vi "ACT_Loop.vi"() -> ()   [LabVIEW 2023, in "SwerveDrive_ACT_ts.lvlib"]
uses:
  SwerveDrive_ACT_ts.lvlib
  Cluster_CMD_ACT_Data.ctl
  Shared Code/TypeDefs/ENUM_CMD_Mode Select.ctl
  Shared Code/TypeDefs/Cluster_CMD_Direction Data.ctl
  Shared Code/TypeDefs/Cluster_Module Velocity-Direction-Rotations.ctl
  Shared Code/TypeDefs/Level_Velocity plus-minus 1.ctl
  Shared Code/TypeDefs/Dial_Compase heading unit circle CCW positive.ctl
  Shared Code/TypeDefs/Cluster_X-Y.ctl
  <vilib>/Rock Robotics/WPI/ThirdParty/REV Robotics/REVLib/Typedef/Spark MAX Control Type.ctl
  Type Defs/ENUM_Steer Mode Select.ctl
  Shared Code/TypeDefs/Cluster_Swerve 4 Steer and Velocity.ctl
  Shared Code/TypeDefs/Cluster_Swerve Actual Settings.ctl
  Shared Code/TypeDefs/Cluster_Module Actual Settings.ctl
  Shared Code/TypeDefs/Dial_Actual Direction.ctl
  ENUM_ACT_State.ctl
  <vilib>/Rock Robotics/WPI/MotorControl/WPI_MotorControlDeviceRef.ctl
  <vilib>/Rock Robotics/WPI/MotorControl/WPI_MotorControlType.ctl
  <vilib>/Rock Robotics/SystemInterfaces/DIO/FPGA_DIOPWMChannel.ctl
  <vilib>/Rock Robotics/WPI/PWM/WPI_PWMDeadband.ctl
  <vilib>/Rock Robotics/SystemInterfaces/DIO/FPGA_DIOChannel.ctl
  Shared Code/TypeDefs/ENUM_Module Position.ctl
  Type Defs/Cluster_Avoid Zone.ctl
  Shared Code/TypeDefs/Cluster_Config_Swerve Drive Parameters.ctl
  Type Defs/Cluster_Length and Width.ctl
  Shared Code/TypeDefs/Cluster_Config_Swerve_Steer Parm.ctl
  Shared Code/TypeDefs/Cluster_Config_Swerve_Drive Param.ctl
  <vilib>/Rock Robotics/WPI/ThirdParty/Phoenix-LabVIEW/CANCoder/Controls/CTRE_Phoenix_CANcoder_DeviceRef.ctl
  ENUM_ACT_Action.ctl
  RoboRIO Utilities/Global_STOP.vi
  Global_CMD_ACT_Data In.vi
  PigeonIMU/Global_SEN_Data Out.vi
  <vilib>/Rock Robotics/WPI/ThirdParty/Phoenix-LabVIEW/CANCoder/Get/CTRE_Phoenix_CANcoder_GetSensorData.vi
  Global_ACT_Data Out.vi
  PigeonIMU/PigeonIMU_SEN_ts.lvlib
panel:
  out "error out 2":errorcluster
  out "error out":errorcluster
  in  "OVERIDE Tab":enum32{"Teleop-Auto", "Move", "Stop"}(tab)
  in  "SEND CMD(Momentry)":bool
  in  "Rotation Reduction 1-0":dbl=0.5
  in  "Orientation Robot(t) Field(f)":bool=TRUE
  in  "Direction":T1 {"Rotate(Yaw) CCW 1 CW -1" scale=1.0..-1.0; "Traverse"."Angle" scale format="%.3f"; "Traverse"."Velocity" scale=-1.0..1.0 scale format="%.1f"}
  in  "Max Translation Speed (ft/sec)":dbl
  out "Cancoder Values":dbl[](array[numeric]) format="%#.6f"
  out "Steer values":dbl[](array[numeric]) format="%.6g"
  out "unit circ Steer values":dbl[](array[numeric]) format="%.6g"
  out "unit circ Cancoder values":dbl[](array[numeric]) format="%#.6f"
  out "Yaw":T4 scale format="%.3f"
  out "Swerve SET Actual":T5 {"Back Right"."Encoder" format="%.2f"; "Back Right"."Direction" scale format="%.3f"; "Back Right"."Velocity" format="%.2f"; "Back Left"."Encoder" format="%.2f"; "Back Left"."Direction" scale format="%.3f"; "Back Left"."Velocity" format="%.2f"; "Front Left"."Encoder" format="%.2f"; "Front Left"."Direction" scale format="%.3f"; "Front Left"."Velocity" format="%.2f"; "Front Right"."Encoder" format="%.2f"; "Front Right"."Direction" scale format="%.3f"; "Front Right"."Velocity" format="%.2f"}
  out "calc time":dbl
  out "Swerve Set":T8 {"Back Right"."Angle" scale format="%.3f"; "Back Right"."Velocity" scale=-1.0..1.0 scale format="%.1f"; "Back Left"."Angle" scale format="%.3f"; "Back Left"."Velocity" scale=-1.0..1.0 scale format="%.1f"; "Front Left"."Angle" scale format="%.3f"; "Front Left"."Velocity" scale=-1.0..1.0 scale format="%.1f"; "Front Right"."Angle" scale format="%.3f"; "Front Right"."Velocity" scale=-1.0..1.0 scale format="%.1f"}
  out "Max Velocity(RPM)":dbl=200.0
  out "Steer Mode":T9
  out "Max Velocity FPS":dbl=2.0
  out "Drive Control Mode":T10
  out "Input CMD":T11 {"Auto Angle" scale format="%.3f"; "Direction"."Rotate(Yaw) CCW 1 CW -1" scale=1.0..-1.0; "Direction"."Traverse"."Angle" scale format="%.3f"; "Direction"."Traverse"."Velocity" scale=-1.0..1.0 scale format="%.1f"}
  out "Cycle Time (S)":dbl format="%.3g"
  # "TeleOp or Auto Control"
  # "STOP"
  # "\"Front\" of Robot"
  # "X"
  # "+CCW"
  # "Y"
  # "(0,0)"
  # "\"Front\" of Robot"
  # "Index 1"
  # "Index 0"
  # "Index 3"
  # "Index 2"
  # "Right Hand Rule"
  # "X"
  # "+CCW"
  # "Y"
  # "(0,0)"
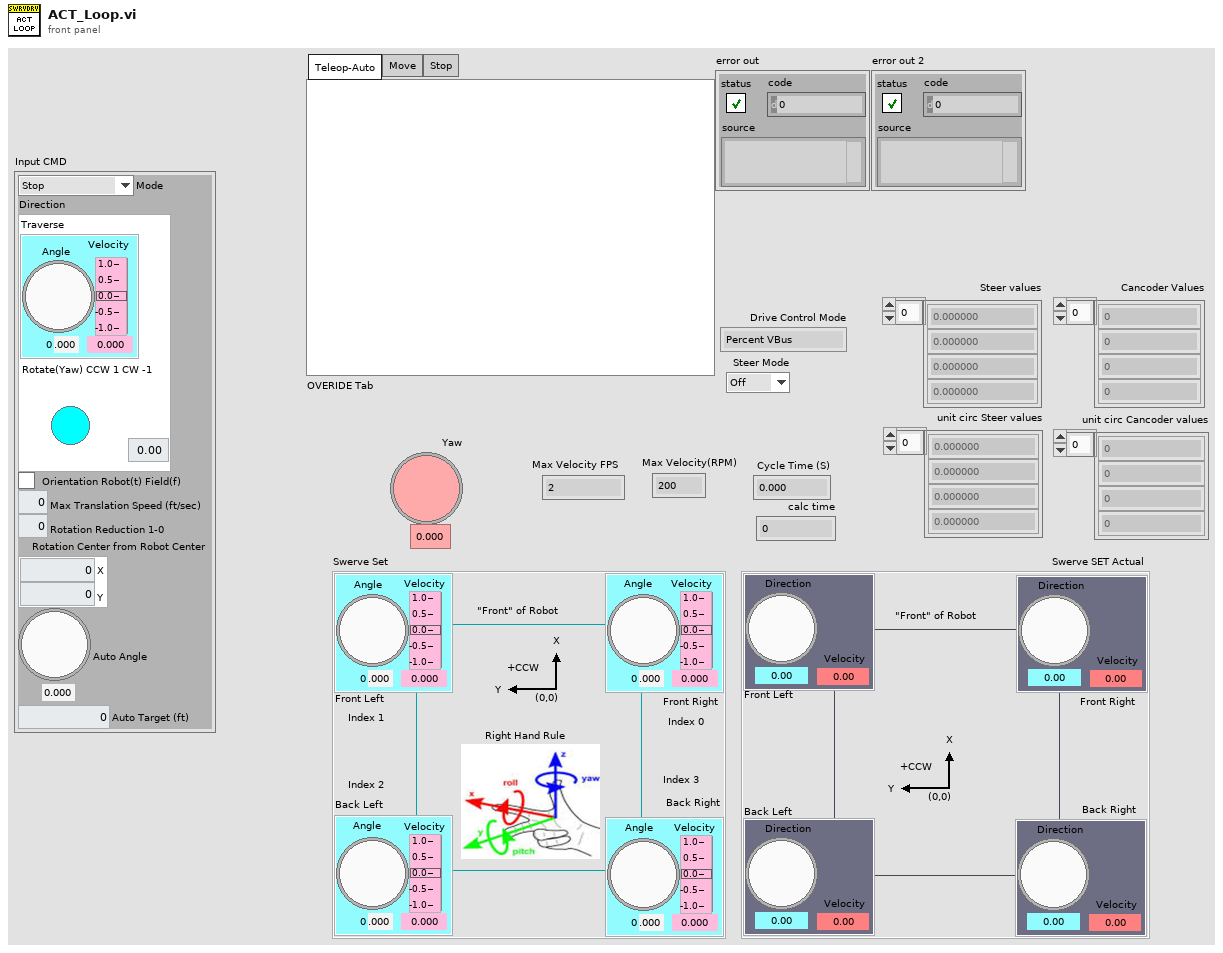
[diagram p1: front panel]
types:
  T1 = typedef "Cluster_CMD_Direction Data.ctl" = cluster{"Traverse":T2, "Rotate(Yaw) CCW 1 CW -1":dbl}
  T2 = typedef "Cluster_Module Velocity-Direction-Rotations.ctl" = cluster{"Velocity":T3, "Angle":T4, "Rotations Count":dbl}
  T3 = typedef "Level_Velocity plus-minus 1.ctl" = dbl
  T4 = typedef "Dial_Compase heading unit circle CCW positive.ctl" = dbl
  T5 = typedef "Cluster_Swerve Actual Settings.ctl" = cluster{"Front Right":T6, "Front Left":T6, "Back Left":T6, "Back Right":T6}
  T6 = typedef "Cluster_Module Actual Settings.ctl" = cluster{"Velocity":dbl, "Direction":T7, "Encoder":dbl}
  T7 = typedef "Dial_Actual Direction.ctl" = dbl
  T8 = typedef "Cluster_Swerve 4 Steer and Velocity.ctl" = cluster{"Front Right":T2, "Front Left":T2, "Back Left":T2, "Back Right":T2}
  T9 = typedef "ENUM_Steer Mode Select.ctl" = enum16{"Off", "Hold", "Steer"}
  T10 = typedef "Spark MAX Control Type.ctl" = enum16{"Percent VBus", "Voltage", "Velocity", "Position", "Smart Motion", "Current", "Smart Velocity"}
  T11 = typedef "SwerveDrive_ACT_ts.lvlib/Cluster_CMD_ACT_Data.ctl" = cluster{"Mode":T12, "Direction":T1, "Orientation Robot(t) Field(f)":bool, "Max Translation Speed (ft/sec)":dbl, "Rotation Reduction 1-0":dbl, "Rotation Center from Robot Center":T13, "Auto Angle":T4, "Auto Target (ft)":dbl}
  T12 = typedef "ENUM_CMD_Mode Select.ctl" = enum16{"Stop", "Move", "Turret Manual"}
  T13 = typedef "Cluster_X-Y.ctl" = cluster{"X":dbl, "Y":dbl}
  T14 = typedef "CTRE_Phoenix_CANcoder_DeviceRef.ctl" = cluster{"DeviceStatus":errorcluster, "Device Number":u8, "Handle":u64, "UsageFrame":u32, "Library Path":path}
  T15 = typedef "Cluster_Config_Swerve Drive Parameters.ctl" = cluster{"SwerveParam Ver":u64, "Frame":T16, "Steer":T17, "Drive":T18}
  T16 = typedef "Cluster_Length and Width.ctl" = cluster{"Length":dbl, "Width":dbl}
  T17 = typedef "Cluster_Config_Swerve_Steer Parm.ctl" = cluster{"CPR":dbl}
  T18 = typedef "Cluster_Config_Swerve_Drive Param.ctl" = cluster{"CPR":dbl, "RevMotor/Wheel":dbl, "Wheel Diameter (in)":dbl}
  T19 = typedef "Cluster_Avoid Zone.ctl" = cluster{"pos 1":dbl, "pos 2":dbl}
  T20 = typedef "ENUM_Module Position.ctl" = enum16{"Left-Front", "Right-Front", "Left-Back", "Right-Back"}
  T21 = typedef "WPI_MotorControlDeviceRef.ctl" = cluster{"DeviceStatus":errorcluster, "Type":T22, "PWM":cluster{"PWM Channel":T23, "DeadBand":T24}, "CAN":cluster{"Device Number":u8, "SetOutput VI Ref":variant, "GetOutput VI Ref":variant, "Enable VI Ref":variant, "Disable VI Ref":variant, "Data":variant}, "Invert":bool, "DIO PWM":cluster{"PWM \"Enable\" Channel":T23, "DIOChannel":T25, "PWM Rate":dbl}}
  T22 = typedef "WPI_MotorControlType.ctl" = enum16{"PWM", "CAN", "DIO PWM"}
  T23 = typedef "FPGA_DIOPWMChannel.ctl" = enum8{"PWM 0", "PWM 1", "PWM 2", "PWM 3", "PWM 4", "PWM 5", "PWM 6", "PWM 7", "PWM 8", "PWM 9", "PWM MXP 0", "PWM MXP 1", "PWM MXP 2", "PWM MXP 3", "PWM MXP 4", "PWM MXP 5", "PWM MXP 6", "PWM MXP 7", "PWM MXP 8", "PWM MXP 9", "Invalid"}
  T24 = typedef "WPI_PWMDeadband.ctl" = cluster{"Name":string, "maxPositivePwm":i32, "minPositivePwm":i32, "centerPwm":i32, "maxNegativePwm":i32, "minNegativePwm":i32, "angularRange":u16}
  T25 = typedef "FPGA_DIOChannel.ctl" = enum8{"DIO 0", "DIO 1", "DIO 2", "DIO 3", "DIO 4", "DIO 5", "DIO 6", "DIO 7", "DIO 8", "DIO 9", "DIO MXP 0", "DIO MXP 1", "DIO MXP 2", "DIO MXP 3", "DIO MXP 4", "DIO MXP 5", "DIO MXP 6", "DIO MXP 7", "DIO MXP 8", "DIO MXP 9", "DIO MXP 10", "DIO MXP 11", "DIO MXP 12", "DIO MXP 13", "DIO MXP 14", "DIO MXP 15", "SPI Port CS1", "SPI Port CS2", "SPI Port CS3", "SPI Port MISO", "SPI Port MOSI", "Invalid"}
  T26 = typedef "SwerveDrive_ACT_ts.lvlib/ENUM_ACT_State.ctl" = enum16{"Startup", "Stopping", "Moving", "Shutdown"}
  T27 = typedef "SwerveDrive_ACT_ts.lvlib/ENUM_ACT_Action.ctl" = enum16{"No Action", "Reset Time", "Reset All", "2 Pos Set Direction", "2 Pos Set Speed", "Record Data", "Set Move from Values", "Reset Steer to Absolute"}
  T28 = cluster{"Motor List":T20[], "Drive Refs":T21[], "Steer Refs":T21[], "State":T26, "Previous State":T26, "Current Time":timestamp, "Previous Time":timestamp, "Start Time":timestamp, "Target Time (ms)":u32, "Cycle Time(S)":dbl, "ACT Input":T11, "Drive Control Mode":T10, "Drive PID Slot":i32, "Steer Position Values":dbl[], "Drive Velocity Values":dbl[], "Steer Position Times":dbl[], "Drive Velocity Times":dbl[], "Stream":bool, "Drive Output Times":dbl[], "Drive Output Values":dbl[], "Zero Start Steer Positions":dbl[], "Steer Mode":T9, "Max Velocity RPM":dbl, "Avoid Zone":T19, "Swerve Set":T8, "calc Start Time":dbl, "Compass Heading":T4, "Swerve Config ":T15, "Team Folder":path, "Steer Output Times":dbl[], "Can Coder Refs":T14[], "Can Coder Output postions":dbl[]}
  T29 = typedef "Cluster_Unity Yaw-Pitch-Roll.ctl" = cluster{"Yaw":T4, "Pitch":T4, "Roll":T4}
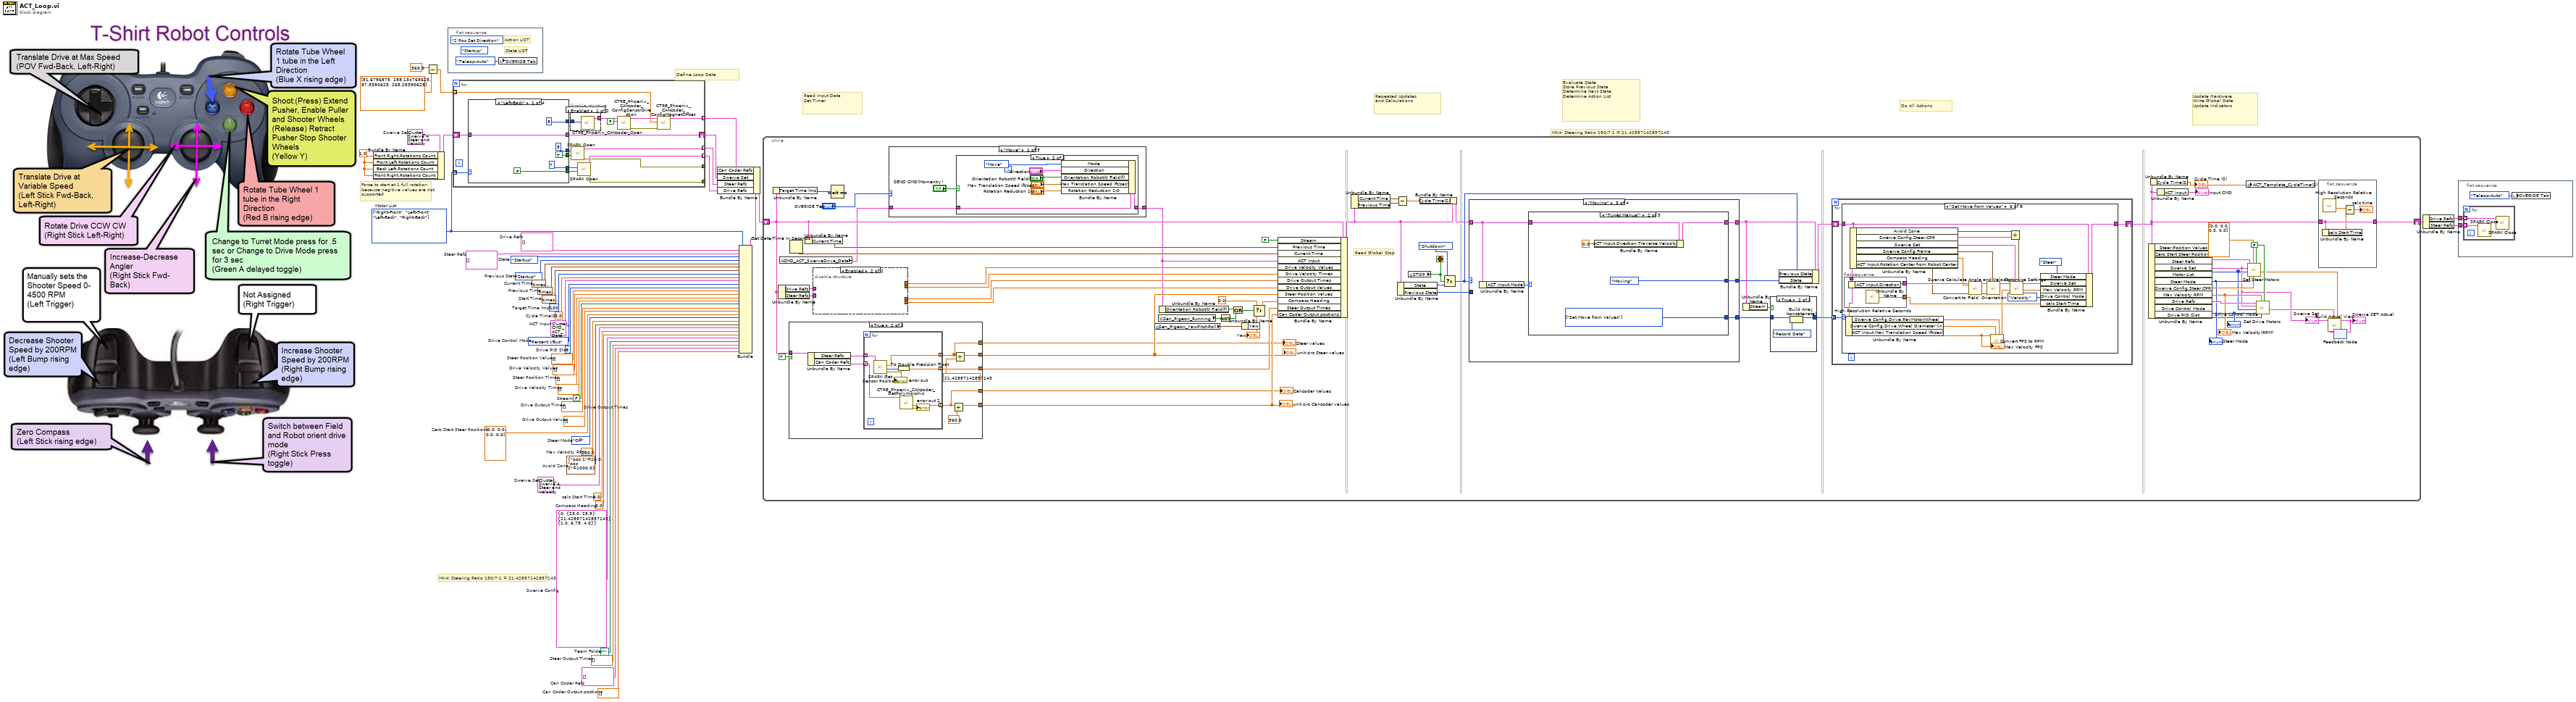
[diagram p0: block diagram]
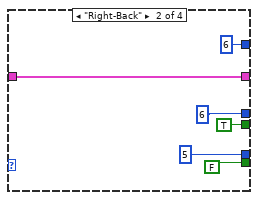
[diagram p3: hidden frame]
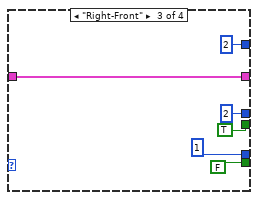
[diagram p4: hidden frame]
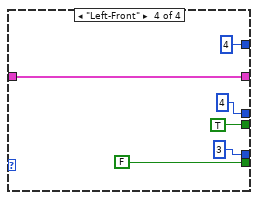
[diagram p5: hidden frame]
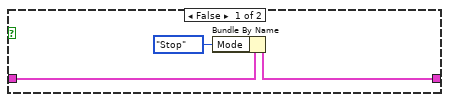
[diagram p6: hidden frame]
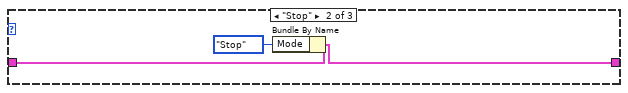
[diagram p7: hidden frame]
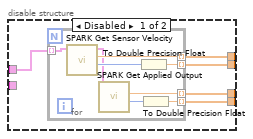
[diagram p9: hidden frame]
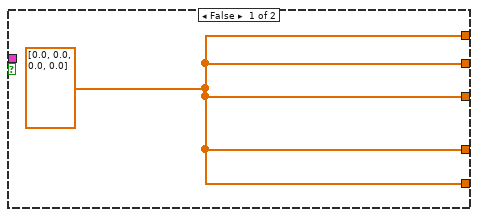
[diagram p10: hidden frame]
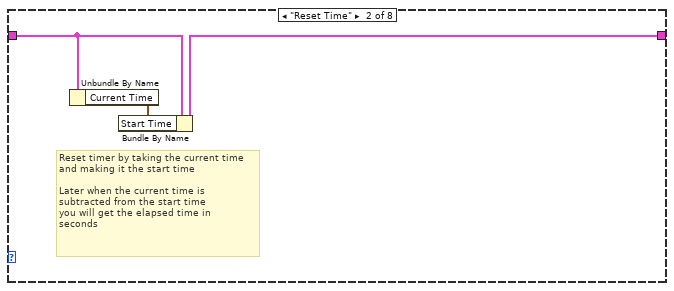
[diagram p13: hidden frame]
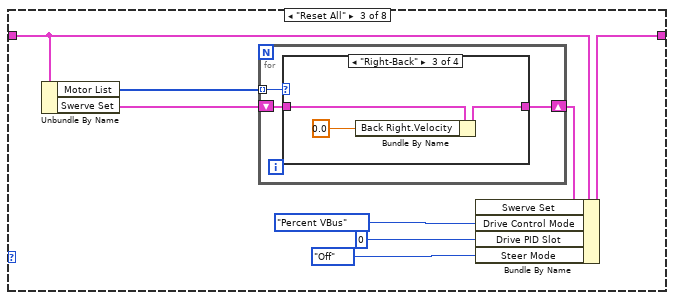
[diagram p14: hidden frame]
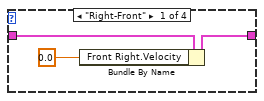
[diagram p15: hidden frame]
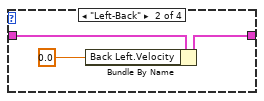
[diagram p16: hidden frame]
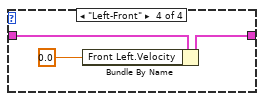
[diagram p17: hidden frame]
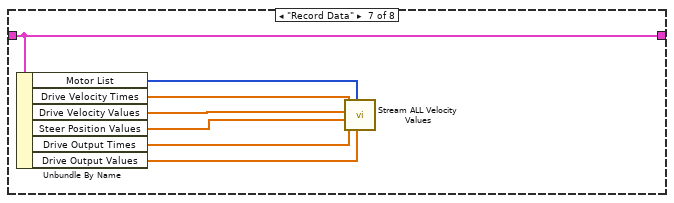
[diagram p20: hidden frame]
diagram:
  w4 = 1.0
  w8 = dbl[] []  # Can Coder Output postions
  w10 = T14[] []  # Can Coder Refs
  w11 = dbl[] []  # Steer Output Times
  (unwired) dbl[] []  # Drive Output Times
  w12 = path ""  # Team Folder
  w13 = T15 {"SwerveParam Ver"=0, "Frame"={"Length"=23.0, "Width"=25.5}, "Steer"={"CPR"=21.42857142857143}, "Drive"={"CPR"=1.0, "RevMotor/Wheel"=6.75, "Wheel Diameter (in)"=4.0}}  # Swerve Config
  w14 = T4 0.0  # Compass Heading
  w15 = 0.0  # calc Start Time
  w6 = T8 {"Front Right"={"Velocity"=0.0, "Angle"=0.0, "Rotations Count"=0.0}, "Front Left"={"Velocity"=0.0, "Angle"=0.0, "Rotations Count"=0.0}, "Back Left"={"Velocity"=0.0, "Angle"=0.0, "Rotations Count"=0.0}, "Back Right"={"Velocity"=0.0, "Angle"=0.0, "Rotations Count"=0.0}}  # Swerve Set
  w17 = T8 {"Front Right"={"Velocity"=0.0, "Angle"=0.0, "Rotations Count"=0.0}, "Front Left"={"Velocity"=0.0, "Angle"=0.0, "Rotations Count"=0.0}, "Back Left"={"Velocity"=0.0, "Angle"=0.0, "Rotations Count"=0.0}, "Back Right"={"Velocity"=0.0, "Angle"=0.0, "Rotations Count"=0.0}}  # Swerve Set
  w18 = T19 {"pos 1"=20.0, "pos 2"=1000.0}  # Avoid Zone
  w19 = T20[] [enum."Right-Front", enum."Left-Front", enum."Left-Back", enum."Right-Back"] items=["Left-Front", "Right-Front", "Left-Back", "Right-Back"]  # Motor List
  w20 = 200.0  # Max Velocity RPM
  w21 = ENUM_Steer_Mode_Select."Off"  # Steer Mode
  w22 = dbl[] [0.0, 0.0, 0.0, 0.0]  # Zero Start Steer Positions
  w23 = dbl[] []  # Drive Output Values
  w24 = dbl[] []  # Drive Output Times
  w25 = FALSE  # Stream
  w26 = dbl[] []  # Drive Velocity Times
  w27 = dbl[] []  # Steer Position Times
  w28 = dbl[] []  # Drive Velocity Values
  w29 = dbl[] []  # Steer Position Values
  w32 = 0  # Drive PID Slot
  w33 = Spark_MAX_Control_Type."Percent VBus"  # Drive Control Mode
  w37 = T21[] []  # Drive Refs
  w38 = T21[] []  # Steer Refs
  w40 = 0.0  # Cycle Time(S)
  w41 = ENUM_ACT_State."Startup"  # Previous State
  w42 = timestamp(0 s since 1904-01-01)  # Previous Time
  w43 = u32 100  # Target Time (ms)
  w44 = T11 {"Mode"=enum."Stop", "Direction"={"Traverse"={"Velocity"=0.0, "Angle"=0.0, "Rotations Count"=0.0}, "Rotate(Yaw) CCW 1 CW -1"=0.0}, "Orientation Robot(t) Field(f)"=FALSE, "Max Translation Speed (ft/sec)"=0.0, "Rotation Reduction 1-0"=0.0, "Rotation Center from Robot Center"={"X"=0.0, "Y"=0.0}, "Auto Angle"=0.0, "Auto Target (ft)"=0.0}  # ACT Input
  w45 = timestamp(0 s since 1904-01-01)  # Start Time
  w46 = timestamp(0 s since 1904-01-01)  # Current Time
  w47 = ENUM_ACT_State."Startup"  # State
  # "Force to start at 1 full rotation\nbecause negitive values are not\nsupported"
  # "MK4i Steering Ratio 150/7:1 = 21.42857142857143"
  # "MK4i Steering Ratio 150/7:1 = 21.42857142857143"
  # "Define Loop Data"
  # "Repeated Updates\nand Calculations"
  # "Read Input Data\nSet Timer"
  # "Evaluate State\nStore Previous State\nDetermine Next State\nDetermine Action List"
  # "Do All Actions"
  # "Update Hardware\nWrite Global Data\nUpdate Indicators"
  n1 = Bundle By Name(cluster=w6, "Front Right.Rotations Count"=w4, "Front Left.Rotations Count"=w4, "Back Left.Rotations Count"=w4, "Front Right.Rotations Count"=w4) -> (w5:T8)
  n2 = Subtract(x=360.0, y=dbl[] [51.6796875, 258.134765625, 87.5390625, 265.25390625] ("Cancoder Values")) -> (x-y=w1:dbl[])
  n3 = flat-sequence {
    frame #0 {
      (unwired) ENUM_ACT_State."Startup" ("State")
      (unwired) ENUM_ACT_Action."2 Pos Set Direction" ("Action")
      # "State LIST"
      # "Action LIST"
      n4 = local write "OVERIDE Tab"(enum32{"Teleop-Auto", "Move", "Stop"}."Teleop-Auto" ("OVERIDE Tab")) -> ()
    }
  }
  n5 = for {
    tunnel: w19 -> [w66] mode=indexing
    tunnel: [w60] -> w7 mode=indexing
    tunnel: [w63] -> w34 mode=indexing
    shift-right: [w64] -> w16
    shift-left: w5 -> [w65]
    tunnel: [w62] -> _
    tunnel: [w51] -> w9 mode=indexing
    tunnel: [w55] -> _
    tunnel: w1 -> [w49] mode=indexing
    n6 = case shown="\"Left-Back\"" w66 {
      tunnel: [FALSE ("Invert") FALSE ("Invert") FALSE ("Invert") FALSE ("Invert")] -> w61
      tunnel: [u8 7 ("unsigned 8bit integer") u8 5 ("unsigned 8bit integer") u8 1 ("unsigned 8bit integer") u8 3 ("unsigned 8bit integer")] -> w59
      tunnel: w65 -> [w69 w75 w81 w87]
      tunnel: [w69 w75 w81 w87] -> w64
      tunnel: [u8 8 ("Device Number") u8 6 ("Device Number") u8 2 ("Device Number") u8 4 ("Device Number")] -> w58
      tunnel: [TRUE ("Invert") TRUE ("Invert") TRUE ("Invert") TRUE ("Invert")] -> w57
      tunnel: [u8 8 ("Device Number") u8 6 ("Device Number") u8 2 ("Device Number") u8 4 ("Device Number")] -> w56
      frame "Left-Back" {
      }
      frame "Right-Back" {
      }
      frame "Right-Front" {
      }
      frame "Left-Front" {
      }
    }
    n7 = disable-structure shown="Enabled" {
      disable-tunnel: [w68 _] -> w54
      disable-tunnel: w56 -> [w67 _]
      frame Enabled {
        n8 = call <vilib>:"CTRE_Phoenix_CANcoder_Open.vi"("Device Number"=w67) -> ("CTRE_CANcoder_DeviceRef"=w68:T14)  [unwired: 9 in, 1 out]
      }
      frame Disabled {
      }
    }
    n9 = call <vilib>:"SPARK Open.vi"("Invert"=w57, "Device Number"=w58) -> ("error out"=w55:errorcluster, "MotorControlDeviceRef"=w60:T21)  [unwired: 8 in]
    n10 = call <vilib>:"SPARK Open.vi"("Invert"=w61, "Device Number"=w59) -> ("error out"=w62:errorcluster, "MotorControlDeviceRef"=w63:T21)  [unwired: 8 in]
    n11 = call <vilib>:"CTRE_Phoenix_CANcoder_ConfigSensorDirection.vi"("Sensor Direction"=FALSE, "CTRE_CANcoder_DeviceRef"=w54) -> ("error out"=w50:errorcluster, "CTRE_CANcoder_DeviceRef"=w52:T14)  [unwired: 8 in]
    n12 = call <vilib>:"CTRE_Phoenix_CANcoder_ConfigMagnetOffset.vi"("error in"=w50, "Magnet Offset (Degrees)"=w49, "CTRE_CANcoder_DeviceRef"=w52) -> ("CTRE_CANcoder_DeviceRef"=w51:T14)  [unwired: 7 in, 1 out]
  }
  n13 = Bundle("Motor List"=w19, "Drive Refs"=w37, "Steer Refs"=w38, "State"=w47, "Previous State"=w41, "Current Time"=w46, "Previous Time"=w42, "Start Time"=w45, "Target Time (ms)"=w43, "Cycle Time(S)"=w40, "ACT Input"=w44, "Drive Control Mode"=w33, "Drive PID Slot"=w32, "Steer Position Values"=w29, "Drive Velocity Values"=w28, "Steer Position Times"=w27, "Drive Velocity Times"=w26, "Stream"=w25, "Drive Output Times"=w24, "Drive Output Values"=w23, "Zero Start Steer Positions"=w22, "Steer Mode"=w21, "Max Velocity RPM"=w20, "Avoid Zone"=w18, "Swerve Set"=w17, "calc Start Time"=w15, "Compass Heading"=w14, "Swerve Config"=w13, "Team Folder"=w12, "Steer Output Times"=w11, "Can Coder Refs"=w10, "Can Coder Output postions"=w8) -> (w36:T28)  [unwired: 1 in]
  n14 = Bundle By Name(cluster=w36, "Can Coder Refs"=w9, "Swerve Set"=w16, "Steer Refs"=w7, "Drive Refs"=w34) -> (w35:T28)
  n15 = while {
    shift-right: [w100] -> w39
    shift-left: w35 -> [w127]
    stop <- w152 stop-if-true
    w116 = FALSE
    # "Read Global Stop"
    n16 = Unbundle By Name(w127) -> ("Target Time (ms)"=w149:u32)
    n17 = Unbundle By Name(w127) -> ("Drive Refs"=w126:T21[], "Steer Refs"=w99:T21[])
    n18 = global read "Global_CMD_ACT_Data In.vi" "CMD_ACT_SwerveDrive_Data"() -> (w96:T11)
    n19 = case shown="True" TRUE {
      tunnel: [w190 w194] -> w102
      tunnel: w127 -> [_ w200]
      tunnel: [w190 w195] -> w101
      tunnel: [w190 w197] -> w103
      tunnel: [w190 w192] -> w98
      tunnel: [w190 w191] -> w97
      frame False {
        w190 = dbl[] [0.0, 0.0, 0.0, 0.0]
      }
      frame True {
        n20 = Unbundle By Name(w200) -> ("Steer Refs"=w198:T21[], "Can Coder Refs"=w199:T14[])
        n21 = for {
          tunnel: [w204] -> w192 mode=indexing
          tunnel: [w207] -> w195 mode=indexing
          tunnel: w199 -> [w203] mode=indexing
          tunnel: [w206] -> w191 mode=indexing
          tunnel: w198 -> [w205] mode=indexing
          n22 = call <vilib>:"SPARK Get Sensor Position.vi"("MotorControlDevRef in"=w205) -> ("error out"=→"error out":errorcluster, "Timestamp"=w208:u32, "Sensor Position"=w204:dbl)  [unwired: 7 in, 1 out]
          n23 = To Double Precision Float(number=w208) -> (double precision float=w207:dbl)
          n24 = call-poly <vilib>:"CTRE_Phoenix_CANcoder_GetPolymorphic.vi"("CTRE_CANcoder_DeviceRef"=w203) -> ("Absolute Position"=w206:dbl, "error out"=→"error out 2":errorcluster)  [unwired: 10 in, 3 out]
        }
        n25 = Divide(x=w191, y=360.0 ("Absolute Position")) -> (x/y=w197:dbl[])
        n26 = Divide(x=w192, y=21.42857142857143 ("Absolute Position")) -> (x/y=w194:dbl[])
      }
    }
    "unit circ Cancoder values" <- w103
    "unit circ Steer values" <- w102
    "Steer values" <- w98
    "Cancoder Values" <- w97
    n27 = Get Date/Time In Seconds() -> (seconds since 1Jan1904=w155:timestamp)
    n28 = Unbundle By Name(w127) -> ("Current Time"=w148:timestamp)
    n29 = disable-structure shown="Enabled" {
      disable-tunnel: [w177 _] -> w136
      disable-tunnel: [w176 _] -> w135
      disable-tunnel: [w175 _] -> w133
      disable-tunnel: [w174 _] -> w132
      disable-tunnel: w126 -> [w173 _]
      disable-tunnel: w99 -> [_ _]
      frame Disabled {
        n30 = for {
          tunnel: w173 -> [w183] mode=indexing
          tunnel: [w182] -> w177 mode=indexing
          tunnel: [w185] -> w176 mode=indexing
          tunnel: [w179] -> w175 mode=indexing
          tunnel: [w184] -> w174 mode=indexing
          n31 = call <vilib>:"SPARK Get Sensor Velocity.vi"("MotorControlDevRef in"=w183) -> ("Timestamp"=w181:u32, "Sensor Velocity"=w182:dbl, "MotorControlDevRef out"=w180:T21)  [unwired: 7 in, 1 out]
          n32 = call <vilib>:"SPARK Get Applied Output.vi"("MotorControlDevRef in"=w180) -> ("Timestamp"=w178:u32, "Applied Output"=w179:dbl)  [unwired: 7 in, 2 out]
          n33 = To Double Precision Float(number=w181) -> (double precision float=w185:dbl)
          n34 = To Double Precision Float(number=w178) -> (double precision float=w184:dbl)
        }
      }
      frame Enabled {
      }
    }
    n35 = Wait (ms)(milliseconds to wait=w149) -> ()  [unwired: 1 out]
    n36 = case shown="\"Move\"" "OVERIDE Tab" {
      tunnel: w96 -> [w157 w171 w172]
      tunnel: [w156 w170 w172] -> w95
      frame "Move" {
        n37 = case shown="True" "SEND CMD(Momentry)" {
          tunnel: w157 -> [w161 w168]
          tunnel: [w160 w167] -> w156
          frame False {
            n38 = Bundle By Name(cluster=w161, "Mode"=ENUM_CMD_Mode_Select."Stop") -> (w160:T11)
          }
          frame True {
            n39 = Bundle By Name(cluster=w168, "Mode"=ENUM_CMD_Mode_Select."Move", "Direction"="Direction", "Orientation Robot(t) Field(f)"="Orientation Robot(t) Field(f)", "Max Translation Speed (ft/sec)"="Max Translation Speed (ft/sec)", "Rotation Reduction 1-0"="Rotation Reduction 1-0") -> (w167:T11)
          }
        }
      }
      frame "Stop" {
        n40 = Bundle By Name(cluster=w171, "Mode"=ENUM_CMD_Mode_Select."Stop") -> (w170:T11)
      }
      frame "Teleop-Auto" {
      }
    }
    n41 = global read "Global_SEN_Data Out.vi" "Sen_Pigeon_YawPitchRoll"() -> (w110:T29)
    n42 = global read "Global_SEN_Data Out.vi" "Sen_Pigeon_Running"() -> (w106:bool)
    n43 = Unbundle By Name(w95) -> ("Orientation Robot(t) Field(f)"=w112:bool)
    n44 = Not(x=w106) -> (.not. x?=w105:bool)
    n45 = Or(x=w112, y=w105) -> (x .or. y?=w107:bool)
    n46 = Unbundle By Name(w110) -> ("Yaw"=w109:T4)
    "Yaw" <- w109
    n47 = Select(t=T4 0.0, s=w107, f=w109) -> (s? t:f=w111:T4)
    n48 = Bundle By Name(cluster=w127, "Stream"=FALSE, "Previous Time"=w148, "Current Time"=w155, "ACT Input"=w95, "Drive Velocity Values"=w136, "Drive Velocity Times"=w135, "Drive Output Times"=w133, "Drive Output Values"=w132, "Steer Position Values"=w102, "Compass Heading"=w111, "Steer Output Times"=w101, "Can Coder Output postions"=w103) -> (w143:T28)
    n49 = Unbundle By Name(w143) -> ("Current Time"=w144:timestamp, "Previous Time"=w145:timestamp)
    n50 = Subtract(x=w144, y=w145) -> (x-y=w141:dbl)
    n51 = Unbundle By Name(w143) -> ("State"=w150:T26, "Previous State"=w147:T26)
    n52 = global read "Global_STOP.vi" "STOP"() -> (w152:bool)
    n53 = Bundle By Name(cluster=w143, "Cycle Time(S)"=w141) -> (w142:T28)
    n54 = Select(t=ENUM_ACT_State."Shutdown" ("State"), s=w152, f=w150) -> (s? t:f=w146:T26)
    n55 = case shown="\"Moving\"" w146 {
      tunnel: w142 -> [w288 w295 w307 w323]
      tunnel: [w290 w296 w308 w323] -> w131
      tunnel: [ENUM_ACT_State."Moving" ("State") w297 w309 ENUM_ACT_State."Shutdown" ("State")] -> w153
      tunnel: [w292 w293 w305 w321] -> w129
      tunnel: w147 -> [_ _ _ _]
      frame "Startup" {
        w292 = T27[] [enum."Reset Steer to Absolute", enum."Reset Time", enum."Reset All", enum."Reset Steer to Absolute"] items=["No Action", "Reset Time", "Reset All", "2 Pos Set Direction", "2 Pos Set Speed", "Record Data", "Set Move from Values", "Reset Steer to Absolute"] ("Actions")
        n56 = Bundle By Name(cluster=w288, "Zero Start Steer Positions"=dbl[] []) -> (w290:T28)
      }
      frame "Stopping" {
        n57 = Unbundle By Name(w295) -> ("ACT Input.Mode"=w294:T12)
        n58 = case shown="\"Stop\"" w294 {
          tunnel: [ENUM_ACT_State."Moving" ("State") ENUM_ACT_State."Moving" ("State") ENUM_ACT_State."Stopping" ("State")] -> w297
          tunnel: [w298 w300 w302] -> w296
          tunnel: w295 -> [w298 w300 w302]
          tunnel: [_ _ w303] -> w293
          frame "Move" {
          }
          frame "Turret Manual" {
          }
          frame "Stop" {
            w303 = T27[] [enum."Reset All", enum."Reset Steer to Absolute"] items=["No Action", "Reset Time", "Reset All", "2 Pos Set Direction", "2 Pos Set Speed", "Record Data", "Set Move from Values", "Reset Steer to Absolute"] ("Actions")
          }
        }
      }
      frame "Moving" {
        n59 = Unbundle By Name(w307) -> ("ACT Input.Mode"=w306:T12)
        n60 = case shown="\"Turret Manual\"" w306 {
          tunnel: [ENUM_ACT_State."Moving" ("State") ENUM_ACT_State."Moving" ("State") ENUM_ACT_State."Stopping" ("State")] -> w309
          tunnel: [w311 w314 w319] -> w308
          tunnel: w307 -> [w311 w313 w319]
          tunnel: [w310 w316 w318] -> w305
          frame "Move" {
            w310 = T27[] [enum."Set Move from Values"] items=["No Action", "Reset Time", "Reset All", "2 Pos Set Direction", "2 Pos Set Speed", "Record Data", "Set Move from Values", "Reset Steer to Absolute"] ("Actions")
          }
          frame "Turret Manual" {
            w316 = T27[] [enum."Set Move from Values"] items=["No Action", "Reset Time", "Reset All", "2 Pos Set Direction", "2 Pos Set Speed", "Record Data", "Set Move from Values", "Reset Steer to Absolute"] ("Actions")
            n61 = Bundle By Name(cluster=w313, "ACT Input.Direction.Traverse.Velocity"=T3 0.0) -> (w314:T28)
          }
          frame "Stop" {
            w318 = T27[] [enum."Reset All"] items=["No Action", "Reset Time", "Reset All", "2 Pos Set Direction", "2 Pos Set Speed", "Record Data", "Set Move from Values", "Reset Steer to Absolute"] ("Actions")
          }
        }
      }
      frame "Shutdown" {
        w321 = T27[] [enum."Reset All"] items=["No Action", "Reset Time", "Reset All", "2 Pos Set Direction", "2 Pos Set Speed", "Record Data", "Set Move from Values", "Reset Steer to Absolute"] ("Actions")
      }
    }
    n62 = Unbundle By Name(w131) -> ("Stream"=w130:bool)
    n63 = case shown="True" w130 {
      tunnel: w129 -> [w209 w212]
      tunnel: [w209 w211] -> w128
      frame False {
      }
      frame True {
        n64 = Build Array (concatenate)(w212, ENUM_ACT_Action."Record Data" ("Action")) -> (w211:T27[])
      }
    }
    n65 = Bundle By Name(cluster=w131, "Previous State"=w146, "State"=w153) -> (w154:T28)
    n66 = for {
      tunnel: w128 -> [w215] mode=indexing
      shift-right: [w214] -> w118
      shift-left: w154 -> [w213]
      n67 = case shown="\"Set Move from Values\"" w215 {
        tunnel: w213 -> [w216 w219 w224 w243 w244 w260 w274 w278]
        tunnel: [w216 w218 w227 w243 w244 w264 w274 w278] -> w214
        frame "No Action" {
        }
        frame "Reset Time" {
          # "Reset timer by taking the current time\nand making it the start time\n\nLater when the current time is \nsubtracted from the start time\nyou will get the elapsed time in \nseconds"
          n68 = Unbundle By Name(w219) -> ("Current Time"=w217:timestamp)
          n69 = Bundle By Name(cluster=w219, "Start Time"=w217) -> (w218:T28)
        }
        frame "Reset All" {
          n70 = Unbundle By Name(w224) -> ("Motor List"=w222:T20[], "Swerve Set"=w221:T8)
          n71 = for {
            tunnel: w222 -> [w230] mode=indexing
            shift-right: [w228] -> w220
            shift-left: w221 -> [w229]
            n72 = case shown="\"Right-Back\"" w230 {
              tunnel: w229 -> [w233 w236 w239 w242]
              tunnel: [w232 w235 w238 w241] -> w228
              frame "Right-Front" {
                n73 = Bundle By Name(cluster=w233, "Front Right.Velocity"=T3 0.0 ("Front Right.Velocity (0-1)")) -> (w232:T8)
              }
              frame "Left-Back" {
                n74 = Bundle By Name(cluster=w236, "Back Left.Velocity"=T3 0.0 ("Front Right.Velocity (0-1)")) -> (w235:T8)
              }
              frame "Right-Back" {
                n75 = Bundle By Name(cluster=w239, "Back Right.Velocity"=T3 0.0 ("Front Right.Velocity (0-1)")) -> (w238:T8)
              }
              frame "Left-Front" {
                n76 = Bundle By Name(cluster=w242, "Front Left.Velocity"=T3 0.0 ("Front Right.Velocity (0-1)")) -> (w241:T8)
              }
            }
          }
          n77 = Bundle By Name(cluster=w224, "Swerve Set"=w220, "Drive Control Mode"=Spark_MAX_Control_Type."Percent VBus", "Drive PID Slot"=0, "Steer Mode"=ENUM_Steer_Mode_Select."Off") -> (w227:T28)
        }
        frame "2 Pos Set Direction" {
        }
        frame "2 Pos Set Speed" {
        }
        frame "Set Move from Values" {
          n78 = flat-sequence {
            tunnel: w260 -> [w267]
            tunnel: [w266] -> w248
            tunnel: [w265] -> w250
            frame #0 {
              n79 = Unbundle By Name(w267) -> ("ACT Input.Direction"=w266:T1)
              n80 = call <vilib>:"High Resolution Relative Seconds.vi"() -> ("relative seconds"=w265:dbl)
            }
          }
          n81 = Unbundle By Name(w260) -> ("Swerve Config.Drive.RevMotor/Wheel"=w258:dbl, "Swerve Config.Drive.Wheel Diameter (in)"=w259:dbl, "ACT Input.Max Translation Speed (ft/sec)"=w246:dbl)
          "Max Velocity FPS" <- w246
          n82 = Unbundle By Name(w260) -> ("Avoid Zone"=w256:T19, "Swerve Config.Steer.CPR"=w257:dbl, "Swerve Set"=w253:T8, "Swerve Config.Frame"=w251:T16, "Compass Heading"=w247:T4, "ACT Input.Rotation Center from Robot Center"=w245:T13)
          n83 = call "Convert to Field  Orientation.vi"("Compass Heading"=w247, "Direction in"=w248) -> ("Corrected Direction out"=w249:T1)  [unwired: 9 in]
          n84 = call "Swerve Calculate Angle and Velocity.vi"("Frame"=w251, "Rotation Center From Robot Center"=w245, "Comand Data"=w249) -> ("Swerve Request Out"=w255:T8)  [unwired: 8 in]
          n85 = call "Convert FPS to RPM.vi"("RevMotor/RevWheel"=w258, "Wheel Diameter (in)"=w259, "Translation Speed (ft/s)"=w246) -> ("Motor Speed (RPM) Out"=w261:dbl)  [unwired: 8 in]
          n86 = Divide(x=w256, y=w257) -> (x/y=w254:T19)
          n87 = call "Optomize Settings.vi"("Aviod Zone"=w254, "Previous Swerve Setting"=w253, "Swerve Request"=w255) -> ("Swerve Setting Out"=w252:T8)  [unwired: 8 in]
          n88 = Bundle By Name(cluster=w260, "Steer Mode"=ENUM_Steer_Mode_Select."Steer", "Swerve Set"=w252, "Max Velocity RPM"=w261, "Drive Control Mode"=Spark_MAX_Control_Type."Velocity", "calc Start Time"=w250) -> (w264:T28)
        }
        frame "Record Data" {
          n89 = Unbundle By Name(w274) -> ("Motor List"=w273:T20[], "Drive Velocity Times"=w272:dbl[], "Drive Velocity Values"=w271:dbl[], "Steer Position Values"=w270:dbl[], "Drive Output Times"=w269:dbl[], "Drive Output Values"=w268:dbl[])
          n90 = call "Stream ALL Velocity Values.vi"("Output Values"=w268, "Motor List"=w273, "Output Times"=w269, "Drive Target Values"=w270, "Drive Velocity Values"=w271, "Drive Times"=w272) -> ()  [unwired: 6 in]
        }
        frame "Reset Steer to Absolute" {
          n91 = Unbundle By Name(w278) -> ("Steer Refs"=w277:T21[], "Can Coder Output postions"=w276:dbl[], "Steer Position Values"=w275:dbl[])
          n92 = for {
            tunnel: w277 -> [w279] mode=indexing
            tunnel: w276 -> [w286] mode=indexing
            tunnel: [w287] -> _
            tunnel: w275 -> [w280] mode=indexing
            w282 = 21.42857142857143 ("Absolute Position")
            # "Convert to Motor Rotations"
            # "Get number of full\n steer rotation"
            n93 = Round Toward -Infinity(1:w280) -> (0:w283:dbl)
            n94 = Multiply(x=w282, y=w283) -> (x*y=w281:dbl)
            n95 = Multiply(x=w286, y=w282) -> (x*y=w285:dbl)
            n96 = Add(x=w285, y=w281) -> (x+y=w284:dbl)
            n97 = call <vilib>:"SPARK Set Sensor Position.vi"("Position"=w284, "MotorControlDeviceRef"=w279) -> ("error out"=w287:errorcluster)  [unwired: 8 in, 1 out]
          }
        }
      }
    }
    n98 = Unbundle By Name(w118) -> ("Steer Refs"=w138:T21[], "Swerve Set"=w104:T8, "Motor List"=w120:T20[], "Steer Mode"=w124:T9, "Swerve Config.Steer.CPR"=w121:dbl, "Max Velocity RPM"=w122:dbl, "Drive Refs"=w137:T21[], "Drive Control Mode"=w123:T10, "Drive PID Slot"=w119:i32)  [unwired: 2 out]
    "Drive Control Mode" <- w123
    "Steer Mode" <- w124
    "Max Velocity(RPM)" <- w122
    "Swerve Set" <- w104
    n99 = Unbundle By Name(w118) -> ("Cycle Time(S)"=w139:dbl)
    "Cycle Time (S)" <- w139
    n100 = Unbundle By Name(w118) -> ("ACT Input"=→"Input CMD":T11)
    n101 = global write "Global_ACT_Data Out.vi" "ACT_Template_CycleTime(S)"(w139) -> ()
    n102 = call "Set Steer Motors.vi"("Disable"=w116, "PPR"=w121, "Offset Encoder Positions"=dbl[] [0.0, 0.0, 0.0, 0.0], "Steer Control Mode"=w124, "Motor List"=w120, "Swerve Data"=w104, "Steer Refs"=w138) -> ("Encoder Counts Out"=w114:dbl[])  [unwired: 3 in, 1 out]
    n103 = call "Set Drive Motors.vi"("Disable"=w116, "Drive PID Slot"=w119, "Max Velocity(RPM)"=w122, "Drive Control Mode"=w123, "Motor List"=w120, "Swerve Data"=w104, "Drive Refs"=w137) -> ("Speeds"=w113:dbl[])  [unwired: 3 in, 1 out]
    n104 = flat-sequence {
      tunnel: w118 -> [w189]
      tunnel: [w189] -> w100
      frame #0 {
        n105 = Unbundle By Name(w189) -> ("calc Start Time"=w187:dbl)
        n106 = call <vilib>:"High Resolution Relative Seconds.vi"() -> ("relative seconds"=w188:dbl)
        n107 = Subtract(x=w188, y=w187) -> (x-y=→"calc time":dbl)
      }
    }
    n108 = feedback #1() -> (w115:T5)  [unwired: 1 in]
    n109 = call "Build Actual View.vi"("Encoder Counts Out"=w114, "Speeds"=w113, "Previous Actual"=w115, "Swerve Set"=w104) -> ("Swerve Data out"=w117:T5)  [unwired: 7 in]
    "Swerve SET Actual" <- w117
    n110 = feedback-in #1(w117) -> ()
  }
  n111 = Unbundle By Name(w39) -> ("Drive Refs"=w30:T21[], "Steer Refs"=w31:T21[])
  n112 = flat-sequence {
    tunnel: w31 -> [w326]
    tunnel: w30 -> [w325]
    frame #0 {
      n113 = for {
        tunnel: w326 -> [w328] mode=indexing
        tunnel: w325 -> [w327] mode=indexing
        n114 = call <vilib>:"SPARK Close.vi"("MotorControlDeviceRef"=w328) -> ()  [unwired: 10 in, 1 out]
        n115 = call <vilib>:"SPARK Close.vi"("MotorControlDeviceRef"=w327) -> ()  [unwired: 10 in, 1 out]
      }
      n116 = local write "OVERIDE Tab"(enum32{"Teleop-Auto", "Move", "Stop"}."Teleop-Auto" ("OVERIDE Tab")) -> ()
    }
  }
